vi "CRYWindow Static Bridge.vi"() -> ()   [LabVIEW 2013]
uses:
  SubVI/CRYMain Sub Window Global.vi
  CRYDocument/CRYReport Global.vi
panel:
  in  "bOpenReportFrame":bool
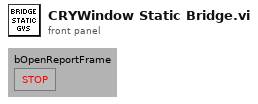
[diagram p1: front panel]
types:
  T1 = cluster{"nID":i32, "sTiltle":string, "pVI":refnum<vi>, "pSP":refnum<vi>, "pTab":refnum<vi>, "pSPT":refnum<vi>, "nWinType":i32, "sIcon":string}
  T2 = cluster{"sAction":string, "sType":string, "sQueueName":string, "sGraphName":string, "sData":string, "nData":i32, "pVIRef":refnum<vi>, "pSPRef":refnum<vi>}
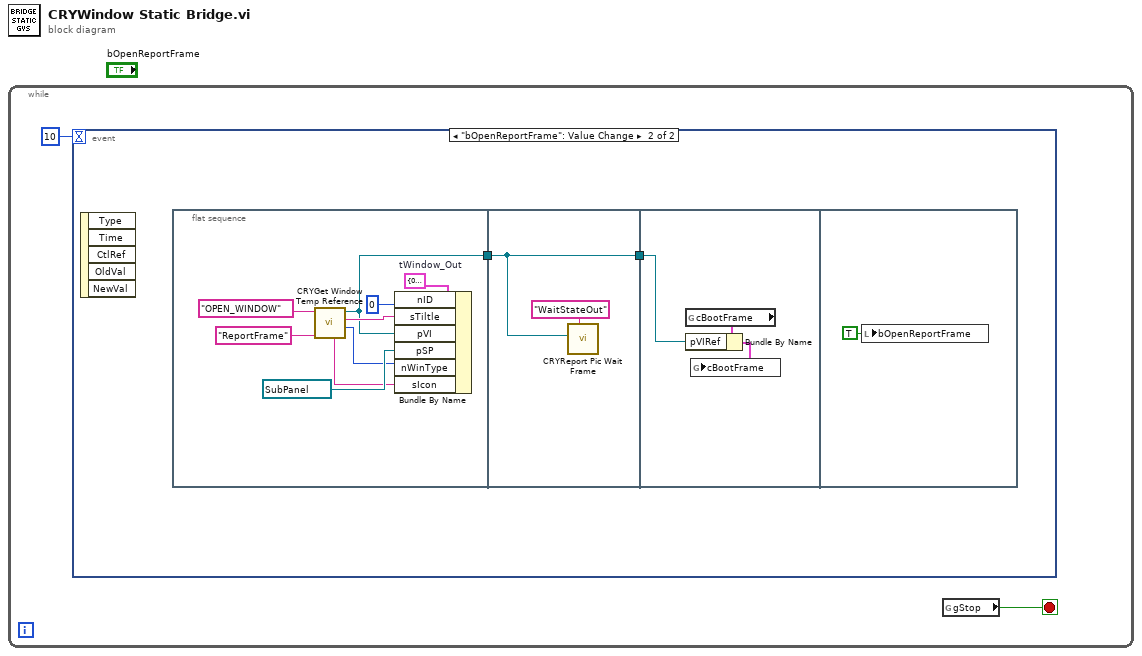
[diagram p0: block diagram]
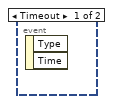
[diagram p2: hidden frame]
diagram:
  n1 = while {
    stop <- w2 stop-if-true
    n2 = event shown="[1] \"bOpenReportFrame\": Value Change" {
      selector: _ -> [_ _]
      dyn-events: _ -> [_ _]
      timeout: 10 -> [_ _]
      event Timeout {
        n3 = event-data() -> ()  [unwired: 1 in, 2 out]
      }
      event "bOpenReportFrame": Value Change {
        n4 = event-data() -> ()  [unwired: 1 in, 5 out]
        n5 = flat-sequence {
          tunnel: [w5] -> w4
          tunnel: w4 -> [w14]
          tunnel: [w14] -> w3
          tunnel: w3 -> [w17]
          frame #0 {
            w13 = T1 {"nID"=0, "sTiltle"="CenterEmpty", "pVI"=refnum, "pSP"=refnum, "pTab"=refnum, "pSPT"=refnum, "nWinType"=0, "sIcon"="CenterEmpty"}  # tWindow_Out
            n6 = call "CRYGet Window Temp Reference.vi"("sWindowName"="ReportFrame" ("sData"), "sAction"="OPEN_WINDOW") -> ("nWinType"=w7:i32, "sTitleName Out"=w8:string, "pVIRef_Out"=w5:refnum<vi>, "sIcon_Out"=w10:string)  [unwired: 2 in, 4 out]
            n7 = Bundle By Name(cluster=w13, "nID"=0, "sTiltle"=w8, "pVI"=w5, "pSP"=refnum<vi> refnum ("pSPRef"), "nWinType"=w7, "sIcon"=w10) -> ()  [unwired: 1 out]
          }
          frame #1 {
            n8 = call "CRYReport Pic Wait Frame.vi"("sAction"="WaitStateOut", "vi reference"=w14) -> ()  [unwired: 9 in, 1 out]
          }
          frame #2 {
            n9 = global read "CRYReport Global.vi" "cBootFrame"() -> (w18:T2)
            n10 = Bundle By Name(cluster=w18, "pVIRef"=w17) -> (w16:T2)
            n11 = global write "CRYReport Global.vi" "cBootFrame"(w16) -> ()
          }
          frame #3 {
            n12 = local write "bOpenReportFrame"(TRUE ("bOpenReportFrame")) -> ()
          }
        }
      }
    }
    n13 = global read "CRYMain Sub Window Global.vi" "gStop"() -> (w2:bool)
  }
